vi "Config Measure Filter.vi"(5 "On/Off (Off)":bool, 6 "Count (1)":i32=1, 7 "Filter Type (Moving Average)":enum32{"Moving Average", "Repeating Average"}(ring), 8 "error in":errorcluster, 9 "Channel (Channel A)":T1, 10 "Node In":string, 11 "VISA resource name":refnum<visa-resource-name>) -> (0 "error out":errorcluster, 2 "Node Out":string, 3 "VISA resource name out":refnum<visa-resource-name>, 4 "Command String":string)   [LabVIEW 2013, in "Keithley 2600 Series.lvlib"]
doc: "This VI configures and enables/disables the measurement filter on the selected SMU.\n\n<b>Functions and Attributes Used</b>\nsmuX.measure.filter.type\nsmuX.measure.filter.count\nsmuX.measure.filter.enable"
uses:
  Keithley 2600 Series.lvlib
  Private/GlobalVariables.vi
  Channel.ctl
panel:
  # "(c) 2008 Keithley Instruments, Inc.  ALL RIGHTS RESERVED."
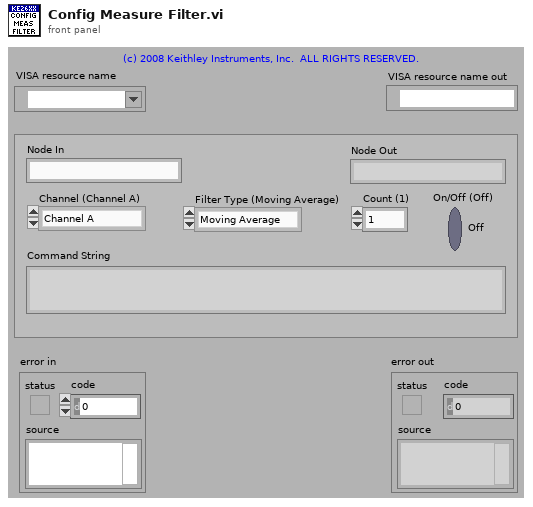
[diagram p1: front panel]
types:
  T1 = typedef "Keithley 2600 Series.lvlib/Channel.ctl" = enum32{"Channel A", "Channel B"}
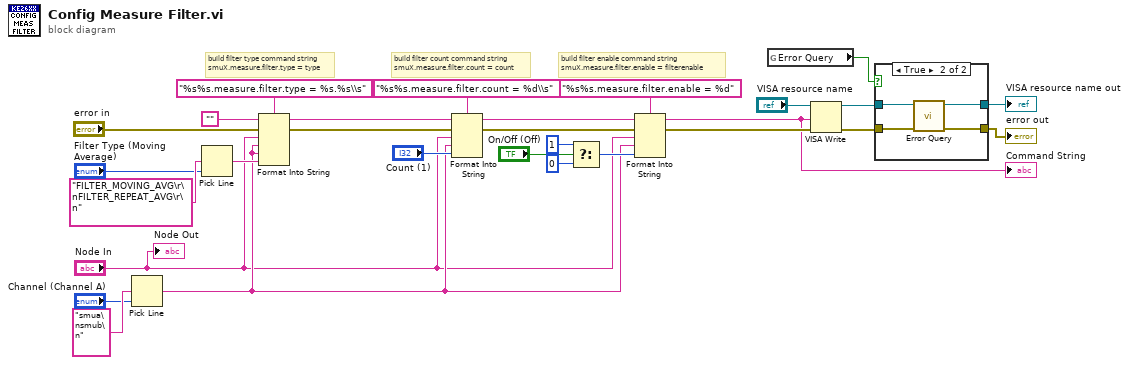
[diagram p0: block diagram]
diagram:
  # "build filter enable command string\nsmuX.measure.filter.enable = filterenable"
  # "build filter count command string\nsmuX.measure.filter.count = count"
  # "build filter type command string\nsmuX.measure.filter.type = type"
  n1 = Pick Line(multi-line string="smua\nsmub\n", line index="Channel (Channel A)") -> (output string=w15:string)  [unwired: 1 out]
  n2 = Pick Line(multi-line string="FILTER_MOVING_AVG\r\nFILTER_REPEAT_AVG\r\n" ("options"), line index="Filter Type (Moving Average)") -> (output string=w24:string)  [unwired: 1 out]
  n3 = Format Into String(format string="%s%s.measure.filter.type = %s.%s\\s", initial string="", error in="error in", "Node In", w15, w15, w24) -> (resulting string=w9:string, error out=w13:errorcluster)
  n4 = Format Into String(format string="%s%s.measure.filter.count = %d\\s", initial string=w9, error in=w13, "Node In", w15, "Count (1)") -> (resulting string=w10:string, error out=w12:errorcluster)
  n5 = Select(t=1, s="On/Off (Off)", f=0) -> (s? t:f=w16:i32)
  n6 = Format Into String(format string="%s%s.measure.filter.enable = %d", initial string=w10, error in=w12, "Node In", w15, w16) -> (resulting string=w1:string, error out=w8:errorcluster)
  "Command String" <- w1
  n7 = global read "GlobalVariables.vi" "Error Query"() -> (w6:bool)
  n8 = VISA Write(VISA resource name="VISA resource name", write buffer=w1, error in (no error)=w8) -> (VISA resource name out=w5:refnum<visa-resource-name>, error out=w4:errorcluster)  [unwired: 1 out]
  n9 = case shown="True" w6 {
    tunnel: w5 -> [w31 w35]
    tunnel: w4 -> [w30 w34]
    tunnel: [w31 w33] -> w3
    tunnel: [w30 w32] -> w2
    frame False {
    }
    frame True {
      n10 = call "Error Query.vi"("error in (no error)"=w34, "VISA resource name"=w35) -> ("error out"=w32:errorcluster, "VISA resource name out"=w33:refnum<visa-resource-name>)  [unwired: 8 out]
    }
  }
  "VISA resource name out" <- w3
  "error out" <- w2
  "Node Out" <- "Node In"
